vi "readt.vi"(10 "Boolean":bool) -> (2 "appended array":dbl[](array[numeric]))   [LabVIEW 2015]
uses:
  <vilib>/Analysis/baseanly.llb/Mean (DBL).vi
  <vilib>/Analysis/NI_AALBase.lvlib
panel:
  out "subarray":dbl[](array[numeric])
  out "Array":dbl[][](array[numeric])
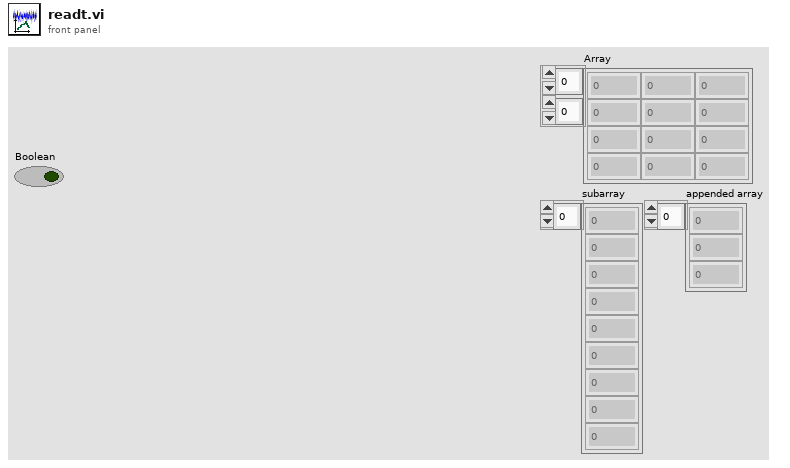
[diagram p1: front panel]
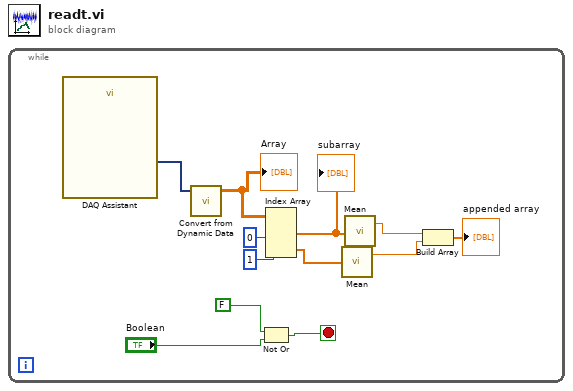
[diagram p0: block diagram]
diagram:
  n1 = while {
    stop <- w1 stop-if-true
    n2 = call "DAQ Assistant"() -> ("data"=w12:dynamicdata)  [unwired: 17 in, 2 out]
    n3 = call "Convert from Dynamic Data"("Dynamic Data Type"=w12) -> ("Array"=w11:dbl[][])  [unwired: 3 in]
    "Array" <- w11
    n4 = Not Or(1:"Boolean", 2:FALSE) -> (0:w1:bool)
    n5 = Index Array(array=w11, index (col) #1=0 ("disabled index (col)"), index (col) #2=1 ("index (col)")) -> (element #1=w10:dbl[], element #2=w7:dbl[])  [unwired: 2 in]
    "subarray" <- w10
    n6 = call-poly <vilib>:"Mean.vi"("X"=w7) -> ("mean"=w5:dbl)  [unwired: 1 out]
    n7 = call-poly <vilib>:"Mean.vi"("X"=w10) -> ("mean"=w6:dbl)  [unwired: 1 out]
    n8 = Build Array(w6, w5) -> (→"appended array":dbl[])
  }
